vi "Ko.vi"(8 "Model":T3=enum."Gallas", 9 "Thermo and Transport Properties":T1, 10 "SJ Geometry":T2, 11 "omega":dbl=0.001) -> (2 "Ko":dbl=2.000052200153926)   [LabVIEW 2012]
uses:
  Model.ctl
  Utilities/fluid_properties/fluid_properties.ctl
  <vilib>/Analysis/2dsp.llb/Integral Method.ctl
  <vilib>/Analysis/8numeric.llb/1D Numeric Integration.vi
  <vilib>/Analysis/1siggen.llb/Ramp Pattern by Samples.vi
  <vilib>/Analysis/1siggen.llb/Ramp Pattern by Delta.vi
  <vilib>/Analysis/NI_AALBase.lvlib
  <vilib>/Analysis/NI_AALPro.lvlib
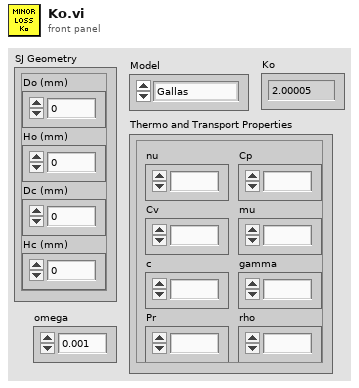
[diagram p1: front panel]
types:
  T1 = typedef "fluid_properties.ctl" = cluster{"nu":dbl, "c":dbl, "Pr":dbl, "Cp":dbl, "Cv":dbl, "gamma":dbl, "mu":dbl, "rho":dbl}
  T2 = cluster{"Do (mm)":dbl, "Ho (mm)":dbl, "Dc (mm)":dbl, "Hc (mm)":dbl}
  T3 = typedef "Model.ctl" = enum16{"Martin", "Tang", "Gallas", "Persoon"}
  T4 = typedef "NI_AALPro.lvlib/Integral Method.ctl" = i32
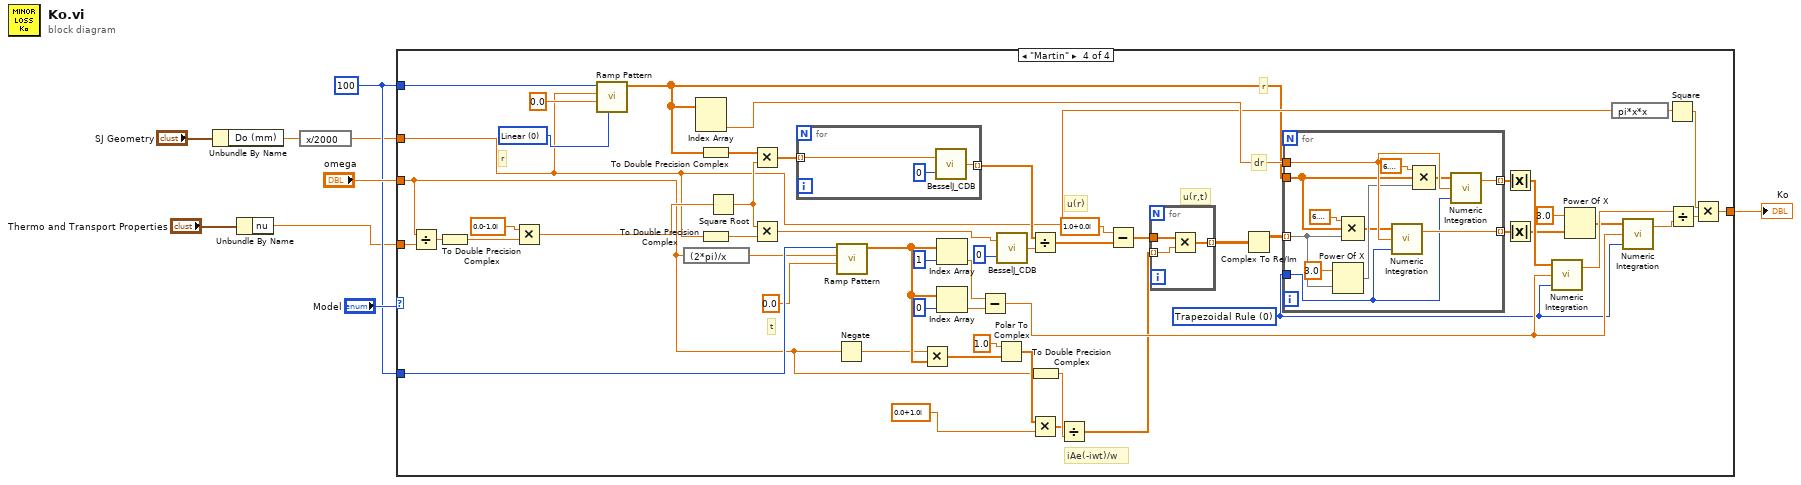
[diagram p0: block diagram]
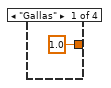
[diagram p2: hidden frame]
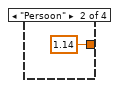
[diagram p3: hidden frame]
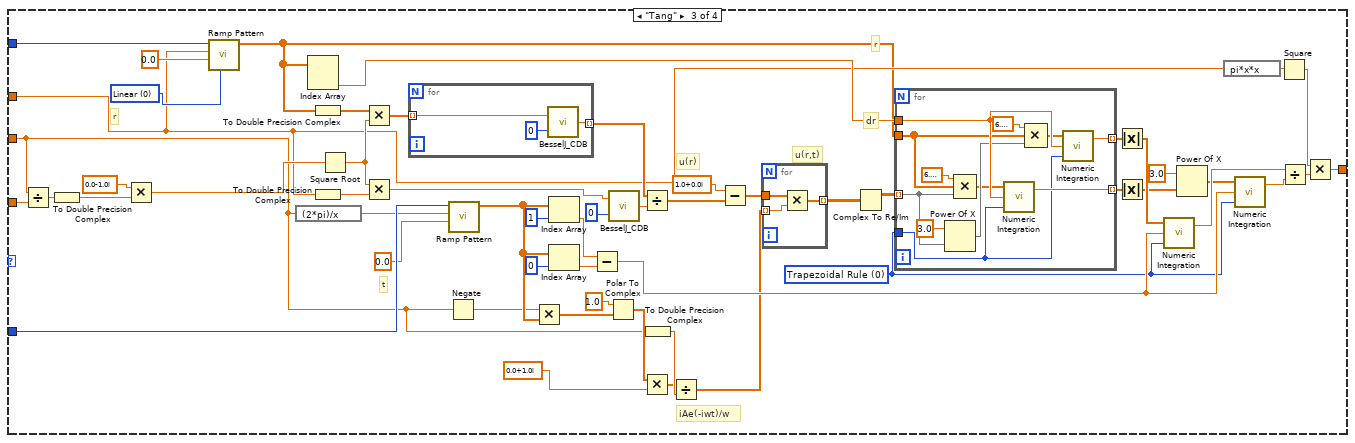
[diagram p4: hidden frame]
diagram:
  w7 = 100 ("n radial pts")
  n1 = Unbundle By Name("SJ Geometry") -> ("Do (mm)"=w5:dbl)
  n2 = Unbundle By Name("Thermo and Transport Properties") -> ("nu"=w2:dbl)
  n3 = expression code="x/2000"(w5) -> (w4:dbl)
  n4 = case shown="\"Martin\"" "Model" {
    tunnel: [1.0 1.14 w66 w139] -> w1
    tunnel: w2 -> [_ _ w51 w124]
    tunnel: w7 -> [_ _ w30 w103]
    tunnel: w7 -> [_ _ w26 w99]
    tunnel: "omega" -> [_ _ w23 w96]
    tunnel: w4 -> [_ _ w21 w94]
    frame "Gallas" {
    }
    frame "Persoon" {
    }
    frame "Tang" {
      w17 = T4 0 items=["Trapezoidal Rule", "Simpson's Rule", "Simpson's 3/8 Rule", "Bode Rule"] ("integration method")
      w27 = u16 0 items=["Linear", "Logarithmic"] ("type")
      # "r"
      # "r"
      # "dr"
      # "u(r)"
      # "u(r,t)"
      # "t"
      # "iAe(-iwt)/w"
      n5 = Divide(x=w23, y=w51) -> (x/y=w52:dbl)
      n6 = To Double Precision Complex(1:w52) -> (0:w53:cdb)
      n7 = Multiply(x=cdb 0.0-1.0i, y=w53) -> (x*y=w54:cdb)
      n8 = call-poly <vilib>:"Ramp Pattern.vi"("type"=w27, "start"=0.0, "end"=w21, "samples"=w26) -> ("Ramp Pattern"=w18:dbl[])  [unwired: 6 in, 1 out]
      n9 = expression code="(2*pi)/x"(w23) -> (w22:dbl)
      n10 = Index Array(array=w18) -> (element #2=w25:dbl)  [unwired: 2 in, 1 out]
      n11 = To Double Precision Complex(1:w18) -> (0:w19:cdb[])
      n12 = To Double Precision Complex(1:w21) -> (0:w24:cdb)
      n13 = Square Root(x=w54) -> (sqrt(x)=w56:cdb)
      n14 = Multiply(x=w19, y=w56) -> (x*y=w55:cdb[])
      n15 = Multiply(x=w56, y=w24) -> (x*y=w14:cdb)
      n16 = for {
        tunnel: w55 -> [w69] mode=indexing
        tunnel: [w67] -> w57 mode=indexing
        n17 = call "BesselJ_CDB.vi"("n"=0, "a+bi"=w69) -> ("Jn(a+bi)"=w67:cdb)
      }
      n18 = Negate(x=w23) -> (-x=w37:dbl)
      n19 = call-poly <vilib>:"Ramp Pattern.vi"("start"=0.0, "end"=w22, "samples"=w30) -> ("Ramp Pattern"=w63:dbl[])  [unwired: 7 in, 1 out]
      n20 = Multiply(x=w37, y=w63) -> (x*y=w35:dbl[])
      n21 = Index Array(array=w63, index=1) -> (element=w40:dbl)
      n22 = Index Array(array=w63, index=0) -> (element=w41:dbl)
      n23 = Subtract(x=w40, y=w41) -> (x-y=w48:dbl)
      n24 = Polar To Complex(1:w35, 2:1.0 ("r")) -> (0:w34:cdb[])
      n25 = call "BesselJ_CDB.vi"("n"=0, "a+bi"=w14) -> ("Jn(a+bi)"=w12:cdb)
      n26 = Divide(x=w57, y=w12) -> (x/y=w58:cdb[])
      n27 = Multiply(x=w34, y=cdb 0.0+1.0i) -> (x*y=w32:cdb[])
      n28 = To Double Precision Complex(1:w23) -> (0:w33:cdb)
      n29 = Divide(x=w32, y=w33) -> (x/y=w36:cdb[])
      n30 = Subtract(x=cdb 1.0+0.0i, y=w58) -> (x-y=w61:cdb[])
      n31 = for {
        tunnel: w61 -> [w84]
        tunnel: w36 -> [w83] mode=indexing
        tunnel: [w82] -> w60 mode=indexing
        n32 = Multiply(x=w84, y=w83) -> (x*y=w82:cdb[])
      }
      n33 = Complex To Re/Im(x + iy=w60) -> (x=w62:dbl[][])  [unwired: 1 out]
      n34 = for {
        tunnel: w62 -> [w72] mode=indexing
        tunnel: w25 -> [w79]
        tunnel: [w80] -> w42 mode=indexing
        tunnel: [w78] -> w44 mode=indexing
        tunnel: w18 -> [w74]
        tunnel: w17 -> [w70]
        n35 = Power Of X(1:w72, 2:3.0) -> (0:w76:dbl[])
        n36 = Compound Arithmetic op=MULTIPLY(6.283185307179586, w74, w72) -> (w71:dbl[])
        n37 = call-poly <vilib>:"Numeric Integration.vi"("integration method"=w70, "dt"=w79, "Input Array"=w71) -> ("result"=w78:dbl)  [unwired: 1 out]
        n38 = Compound Arithmetic op=MULTIPLY(6.283185307179586, w74, w76) -> (w75:dbl[])
        n39 = call-poly <vilib>:"Numeric Integration.vi"("integration method"=w70, "dt"=w79, "Input Array"=w75) -> ("result"=w80:dbl)  [unwired: 1 out]
      }
      n40 = Absolute Value(x=w42) -> (abs(x)=w46:dbl[])
      n41 = Absolute Value(x=w44) -> (abs(x)=w45:dbl[])
      n42 = call-poly <vilib>:"Numeric Integration.vi"("integration method"=w17, "dt"=w48, "Input Array"=w46) -> ("result"=w49:dbl)  [unwired: 1 out]
      n43 = Power Of X(1:w45, 2:3.0) -> (0:w47:dbl[])
      n44 = expression code="pi*x*x"(w21) -> (w20:dbl)
      n45 = call-poly <vilib>:"Numeric Integration.vi"("integration method"=w17, "dt"=w48, "Input Array"=w47) -> ("result"=w64:dbl)  [unwired: 1 out]
      n46 = Square(x=w20) -> (x^2=w16:dbl)
      n47 = Divide(x=w49, y=w64) -> (x/y=w65:dbl)
      n48 = Multiply(x=w16, y=w65) -> (x*y=w66:dbl)
    }
    frame "Martin" {
      w90 = T4 0 items=["Trapezoidal Rule", "Simpson's Rule", "Simpson's 3/8 Rule", "Bode Rule"] ("integration method")
      w100 = u16 0 items=["Linear", "Logarithmic"] ("type")
      # "r"
      # "r"
      # "dr"
      # "u(r)"
      # "u(r,t)"
      # "t"
      # "iAe(-iwt)/w"
      n49 = Divide(x=w96, y=w124) -> (x/y=w125:dbl)
      n50 = To Double Precision Complex(1:w125) -> (0:w126:cdb)
      n51 = Multiply(x=cdb 0.0-1.0i, y=w126) -> (x*y=w127:cdb)
      n52 = call-poly <vilib>:"Ramp Pattern.vi"("type"=w100, "start"=0.0, "end"=w94, "samples"=w99) -> ("Ramp Pattern"=w91:dbl[])  [unwired: 6 in, 1 out]
      n53 = expression code="(2*pi)/x"(w96) -> (w95:dbl)
      n54 = Index Array(array=w91) -> (element #2=w98:dbl)  [unwired: 2 in, 1 out]
      n55 = To Double Precision Complex(1:w91) -> (0:w92:cdb[])
      n56 = To Double Precision Complex(1:w94) -> (0:w97:cdb)
      n57 = Square Root(x=w127) -> (sqrt(x)=w129:cdb)
      n58 = Multiply(x=w92, y=w129) -> (x*y=w128:cdb[])
      n59 = Multiply(x=w129, y=w97) -> (x*y=w87:cdb)
      n60 = for {
        tunnel: w128 -> [w142] mode=indexing
        tunnel: [w140] -> w130 mode=indexing
        n61 = call "BesselJ_CDB.vi"("n"=0, "a+bi"=w142) -> ("Jn(a+bi)"=w140:cdb)
      }
      n62 = Negate(x=w96) -> (-x=w110:dbl)
      n63 = call-poly <vilib>:"Ramp Pattern.vi"("start"=0.0, "end"=w95, "samples"=w103) -> ("Ramp Pattern"=w136:dbl[])  [unwired: 7 in, 1 out]
      n64 = Multiply(x=w110, y=w136) -> (x*y=w108:dbl[])
      n65 = Index Array(array=w136, index=1) -> (element=w113:dbl)
      n66 = Index Array(array=w136, index=0) -> (element=w114:dbl)
      n67 = Subtract(x=w113, y=w114) -> (x-y=w121:dbl)
      n68 = Polar To Complex(1:w108, 2:1.0 ("r")) -> (0:w107:cdb[])
      n69 = call "BesselJ_CDB.vi"("n"=0, "a+bi"=w87) -> ("Jn(a+bi)"=w85:cdb)
      n70 = Divide(x=w130, y=w85) -> (x/y=w131:cdb[])
      n71 = Multiply(x=w107, y=cdb 0.0+1.0i) -> (x*y=w105:cdb[])
      n72 = To Double Precision Complex(1:w96) -> (0:w106:cdb)
      n73 = Divide(x=w105, y=w106) -> (x/y=w109:cdb[])
      n74 = Subtract(x=cdb 1.0+0.0i, y=w131) -> (x-y=w134:cdb[])
      n75 = for {
        tunnel: w134 -> [w157]
        tunnel: w109 -> [w156] mode=indexing
        tunnel: [w155] -> w133 mode=indexing
        n76 = Multiply(x=w157, y=w156) -> (x*y=w155:cdb[])
      }
      n77 = Complex To Re/Im(x + iy=w133) -> (x=w135:dbl[][])  [unwired: 1 out]
      n78 = for {
        tunnel: w135 -> [w145] mode=indexing
        tunnel: w98 -> [w152]
        tunnel: [w153] -> w115 mode=indexing
        tunnel: [w151] -> w117 mode=indexing
        tunnel: w91 -> [w147]
        tunnel: w90 -> [w143]
        n79 = Power Of X(1:w145, 2:3.0) -> (0:w149:dbl[])
        n80 = Compound Arithmetic op=MULTIPLY(6.283185307179586, w147, w145) -> (w144:dbl[])
        n81 = call-poly <vilib>:"Numeric Integration.vi"("integration method"=w143, "dt"=w152, "Input Array"=w144) -> ("result"=w151:dbl)  [unwired: 1 out]
        n82 = Compound Arithmetic op=MULTIPLY(6.283185307179586, w147, w149) -> (w148:dbl[])
        n83 = call-poly <vilib>:"Numeric Integration.vi"("integration method"=w143, "dt"=w152, "Input Array"=w148) -> ("result"=w153:dbl)  [unwired: 1 out]
      }
      n84 = Absolute Value(x=w115) -> (abs(x)=w119:dbl[])
      n85 = Absolute Value(x=w117) -> (abs(x)=w118:dbl[])
      n86 = call-poly <vilib>:"Numeric Integration.vi"("integration method"=w90, "dt"=w121, "Input Array"=w119) -> ("result"=w122:dbl)  [unwired: 1 out]
      n87 = Power Of X(1:w118, 2:3.0) -> (0:w120:dbl[])
      n88 = expression code="pi*x*x"(w94) -> (w93:dbl)
      n89 = call-poly <vilib>:"Numeric Integration.vi"("integration method"=w90, "dt"=w121, "Input Array"=w120) -> ("result"=w137:dbl)  [unwired: 1 out]
      n90 = Square(x=w93) -> (x^2=w89:dbl)
      n91 = Divide(x=w122, y=w137) -> (x/y=w138:dbl)
      n92 = Multiply(x=w89, y=w138) -> (x*y=w139:dbl)
    }
  }
  "Ko" <- w1
